vi "Set Max Retries.vi"(8 "error in":errorcluster, 10 "Max Retries":u8=3, 11 "SDO Manager in":refnum<class "SDO Manager.lvclass">) -> (0 "error out":errorcluster, 3 "SDO Manager out":refnum<class "SDO Manager.lvclass">)   [LabVIEW 2020, in "CANopen.lvlib" / "SDO Manager.lvlib" / "SDO Manager.lvclass"]
uses:
  SDO Manager.lvclass
  SDO Manager.lvclass/SDO Manager.ctl
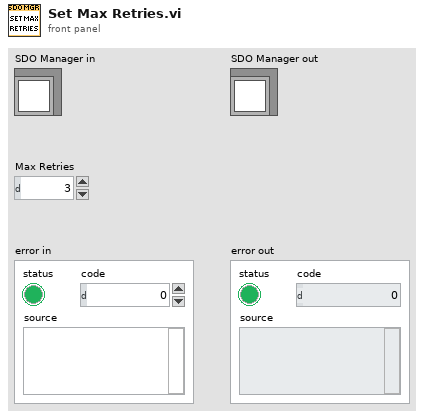
[diagram p1: front panel]
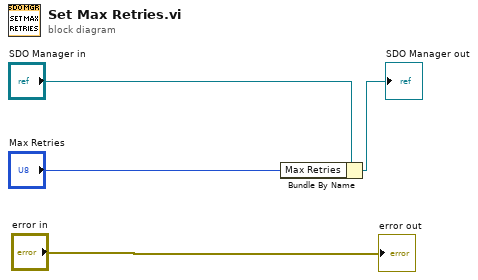
[diagram p0: block diagram]
diagram:
  n1 = Bundle By Name(cluster="SDO Manager in", "Max Retries"="Max Retries") -> (→"SDO Manager out":refnum<class "SDO Manager.lvclass">)
  "error out" <- "error in"
